vi "show_all_Fotos_A.vi"() -> ()   [LabVIEW 2017]
panel:
  in  "#millisecond / foto":dbl(slide)=497.6744186046512 scale=0.0..1000.0
  out "Tot.#Fotos":i32
  out "Boolean Round":bool
  in  "Power On Button":bool
  out "#Foto":i32
  out "imagePath":path
  in  "Folder":path=path "C:/Imagenes/experimentos"
  out "Resized Picture":picture
  # "Lector de imágenes"
  # "asslcdms Feb2023 LV17"
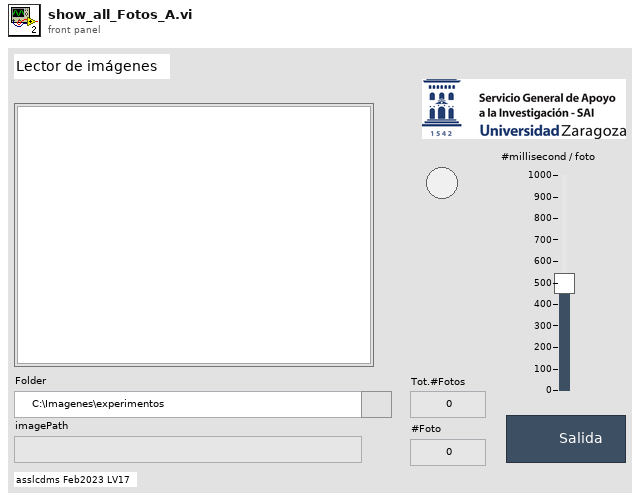
[diagram p1: front panel]
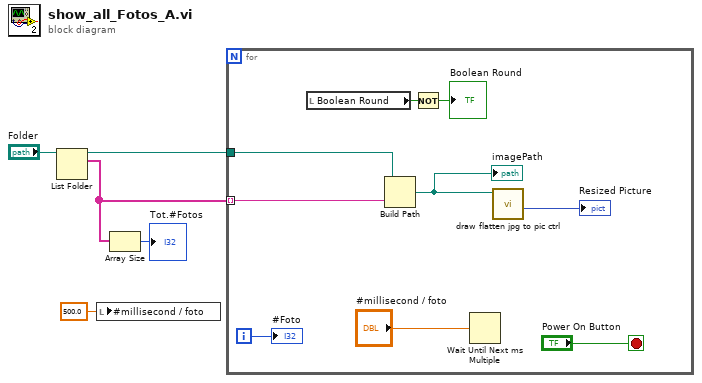
[diagram p0: block diagram]
diagram:
  n1 = List Folder(path="Folder") -> (path out=w4:path, filenames=w3:string[])  [unwired: 3 in, 2 out]
  n2 = local write "#millisecond / foto"(500.0 ("#millisecond / foto")) -> ()
  n3 = Array Size(array=w3) -> (size(s)=→"Tot.#Fotos":i32)
  n4 = for {
    tunnel: w4 -> [w14]
    tunnel: w3 -> [w13] mode=indexing
    i -> [w10]
    stop <- "Power On Button" stop-if-true
    n5 = local read "Boolean Round"() -> (w9:bool)
    n6 = Build Path(base path=w14, name or relative path=w13) -> (appended path=w12:path)
    "imagePath" <- w12
    n7 = Not(x=w9) -> (.not. x?=→"Boolean Round":bool)
    n8 = Wait Until Next ms Multiple(millisecond multiple="#millisecond / foto") -> ()  [unwired: 1 out]
    n9 = call "draw flatten jpg to pic ctrl.vi"("path to JPEG file"=w12) -> ("Picture"=→"Resized Picture":picture)  [unwired: 9 in, 1 out]
    "#Foto" <- w10
  }
